vi "VIPM_Identify New and Modified Spec Files.vi"(7 "Force Reload?(F)":bool, 8 "error in (no error)":errorcluster, 11 "Spec Files":path[](array[path])) -> (0 "error out":errorcluster, 1 "Version map":map{string, i32[]}(c390), 2 "New or Modified Spec Files":path[](array[path]), 3 "Unchanged Package Array":T1[](array[typedef]))   [LabVIEW 2019, in "Project.Dependencies Finder.lvlib" / "Dependency Source_VIPM.lvclass"]
uses:
  Dependency Source_VIPM.lvclass
  Ctl/Ctl_Package Identifier Cluster.ctl
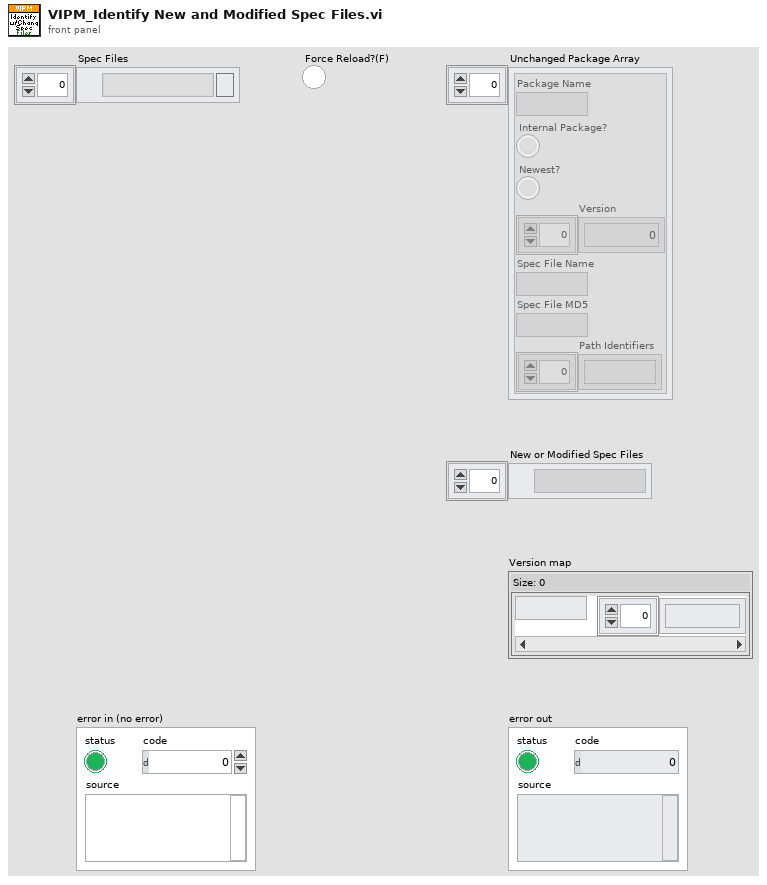
[diagram p1: front panel]
types:
  T1 = typedef "Project.Dependencies Finder.lvlib/Dependency Source_VIPM.lvclass/Ctl_Package Identifier Cluster.ctl" = cluster{"Package Name":string, "Internal Package?":bool, "Newest?":bool, "Version":i32[], "Spec File Name":string, "Spec File MD5":string, "Path Identifiers":string[]}
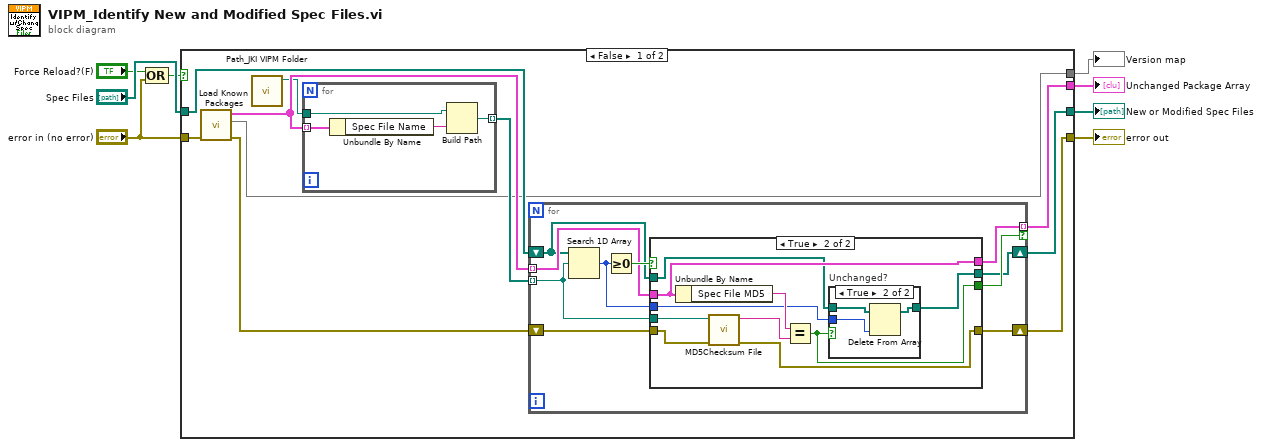
[diagram p0: block diagram]
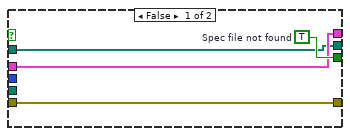
[diagram p2: hidden frame]
diagram:
  n1 = Compound Arithmetic op=OR("Force Reload?(F)", "error in (no error)") -> (w4:bool)
  n2 = case shown="False" w4 {
    tunnel: "Spec Files" -> [w15 w52]
    tunnel: [w14 _] -> w7
    tunnel: [w13 w52] -> w6
    tunnel: [w11 w51] -> w5
    tunnel: "error in (no error)" -> [w10 w51]
    tunnel: [w9 _] -> w1
    frame False {
      n3 = call "Load Known Packages.vi"("error in (no error)"=w10) -> ("error out"=w12:errorcluster, "Version map"=w9:map{string, i32[]}, "Package Array from File"=w18:T1[])  [unwired: 7 in, 1 out]
      n4 = call "Path_JKI VIPM Folder.vi"() -> ("JKI\\VIPM path"=w16:path)  [unwired: 10 in, 1 out]
      n5 = for {
        tunnel: w18 -> [w22] mode=indexing
        tunnel: [w19] -> w17 mode=indexing
        tunnel: w16 -> [w21]
        n6 = Unbundle By Name(w22) -> ("Spec File Name"=w20:string)
        n7 = Build Path(base path=w21, name or relative path=w20) -> (appended path=w19:path)
      }
      n8 = for {
        tunnel: w17 -> [w29] mode=indexing
        tunnel: w18 -> [w28] mode=indexing
        shift-right: [w25] -> w13
        shift-left: w15 -> [w26]
        tunnel: [w27] -> w14 mode=indexing if=w31
        shift-right: [w23] -> w11
        shift-left: w12 -> [w24]
        n9 = Search 1D Array(1D array=w26, element=w29) -> (index of element=w30:i32)  [unwired: 1 in]
        n10 = Greater Or Equal To 0?(x=w30) -> (x >= 0?=w32:bool)
        n11 = case shown="True" w32 {
          tunnel: [w36 w42] -> w31
          tunnel: w30 -> [_ w40]
          tunnel: w29 -> [_ w46]
          tunnel: w28 -> [w35 w43]
          tunnel: [w35 w43] -> w27
          tunnel: w26 -> [w34 w41]
          tunnel: [w34 w39] -> w25
          tunnel: w24 -> [w33 w38]
          tunnel: [w33 w37] -> w23
          frame False {
            w36 = TRUE  # Spec file not found
          }
          frame True {
            n12 = Unbundle By Name(w43) -> ("Spec File MD5"=w44:string)
            n13 = call <vilib>:"MD5Checksum File.vi"("error in (no error)"=w38, "Path"=w46) -> ("error out"=w37:errorcluster, "MD5 message-digest"=w45:string)  [unwired: 8 in]
            n14 = Equal?(x=w44, y=w45) -> (x = y?=w42:bool)
            n15 = case "Unchanged?" shown="True" w42 {
              tunnel: w41 -> [w47 w50]
              tunnel: w40 -> [_ w49]
              tunnel: [w47 w48] -> w39
              frame False {
              }
              frame True {
                n16 = Delete From Array(array=w50, index=w49) -> (array with subset deleted=w48:path[])  [unwired: 1 in, 1 out]
              }
            }
          }
        }
      }
    }
    frame True {
    }
  }
  "error out" <- w5
  "Unchanged Package Array" <- w7
  "New or Modified Spec Files" <- w6
  "Version map" <- w1
